vi "Record Call.vi"(8 "error in (no error)":errorcluster, 10 "VI Call":refnum<class "VI Call.lvclass">, 11 "One Of In":refnum<class "One or More.lvclass">) -> (0 "error out":errorcluster, 3 "One Of Out":refnum<class "One or More.lvclass">)   [LabVIEW 2020, in "One or More.lvclass"]
uses:
  One or More.lvclass
  Call/VI Call.lvclass
  One or More.lvclass/One or More.ctl
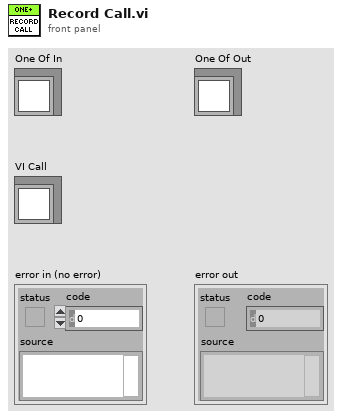
[diagram p1: front panel]
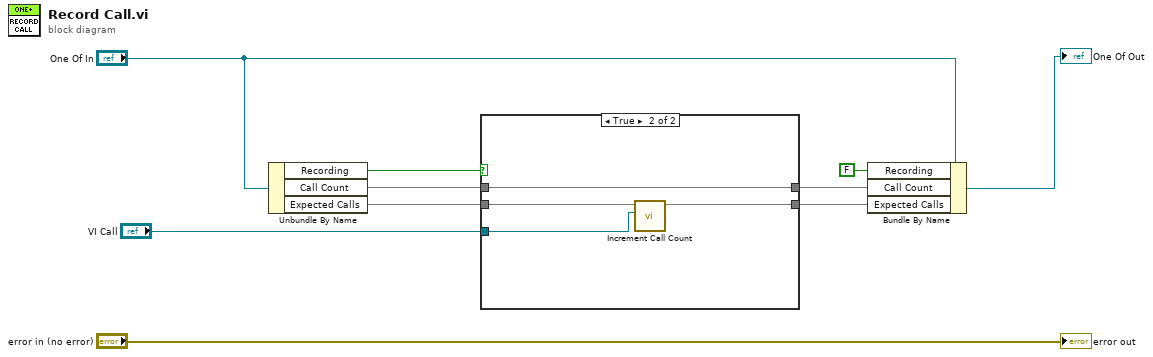
[diagram p0: block diagram]
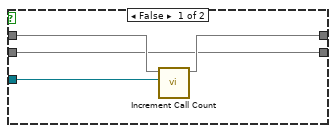
[diagram p2: hidden frame]
diagram:
  n1 = Unbundle By Name("One Of In") -> ("Recording"=w5:bool, "Call Count"=w9:map{refnum<class "VI Call.lvclass">, i32}, "Expected Calls"=w3:map{refnum<class "VI Call.lvclass">, i32})
  n2 = case shown="True" w5 {
    tunnel: w9 -> [w14 w18]
    tunnel: [w13 w18] -> w8
    tunnel: "VI Call" -> [w11 w15]
    tunnel: w3 -> [w12 w17]
    tunnel: [w12 w16] -> w1
    frame False {
      n3 = call "Increment Call Count.vi"("Call in"=w11, "Expected Calls in"=w14) -> ("Expected Calls out"=w13:map{refnum<class "VI Call.lvclass">, i32})  [unwired: 9 in]
    }
    frame True {
      n4 = call "Increment Call Count.vi"("Call in"=w15, "Expected Calls in"=w17) -> ("Expected Calls out"=w16:map{refnum<class "VI Call.lvclass">, i32})  [unwired: 9 in]
    }
  }
  n5 = Bundle By Name(cluster="One Of In", "Recording"=FALSE, "Call Count"=w8, "Expected Calls"=w1) -> (→"One Of Out":refnum<class "One or More.lvclass">)
  "error out" <- "error in (no error)"
